vi "General setup bundler-Boolean.vi"(8 "error in (no error)":errorcluster, 9 "Boolean":T2, 10 "Section":string, 11 "Setup.ini ref":T1) -> (0 "error out":errorcluster, 3 "Setup.ini ref":T1)   [LabVIEW 2013]
uses:
  Typedefs/Ini file interface (Boolean).ctl
  <vilib>/Utility/config.llb/Config Data RefNum.ctl
  <vilib>/Utility/config.llb/NI_LVConfig.lvlib
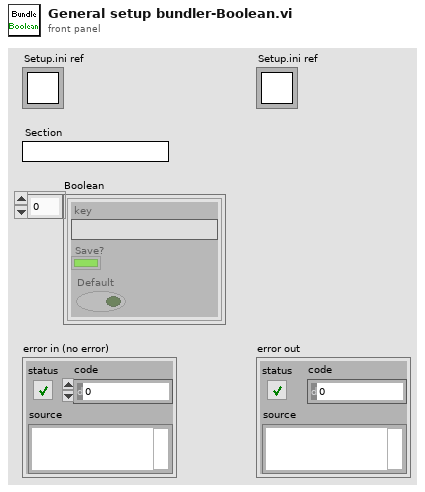
[diagram p1: front panel]
types:
  T1 = typedef "NI_LVConfig.lvlib/Config Data RefNum.ctl" = refnum<k1>
  T2 = typedef "Ini file interface (Boolean).ctl" = cluster{"key":string, "Save?":bool, "Default":bool}[]
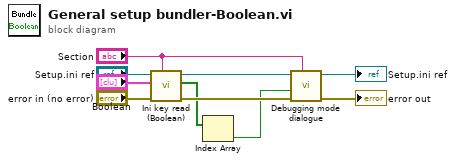
[diagram p0: block diagram]
diagram:
  n1 = call "Ini key read (Boolean).vi"("Section"="Section", "error in (no error)"="error in (no error)", "Parameter names & setup"="Boolean", "Ini file refnum in"="Setup.ini ref") -> ("error out"=→"error out":errorcluster, "Value read/used"=w6:bool[], "Ini file refnum out"=w4:T1)  [unwired: 5 in]
  n2 = Index Array(array=w6) -> (element=w2:bool)  [unwired: 1 in]
  n3 = call "Debugging mode dialogue.vi"("Section"="Section", "Loaded value for \"DevPC - No hardware\""=w2, "Setup.ini ref"=w4) -> ("Setup.ini ref"=→"Setup.ini ref":T1)  [unwired: 8 in]
